vi "basic-speaker.vi"(4 "Cluster":T2, 5 "Period":i64, 6 "Cluster 2":T1, 7 "Lickometer":refnum<vi>, 9 "Speaker in":refnum<vi>, 10 "reference":refnum<vi>, 11 "Cluster in":refnum<vi>) -> (3 "Cluster 3":T1)   [LabVIEW 2015]
uses:
  Device/Methods/Speaker-Play.vi
  <vilib>/Platform/TimedLoop/XDataNode/wakeup.ctl
  <vilib>/Platform/TimedLoop/XDataNode/XDNodeRunTimeDep.lvlib
  <vilib>/Platform/TimedLoop/XDataNode/nitl_modes.ctl
  <vilib>/Platform/TimedLoop/XDataNode/timing_clust.ctl
  <vilib>/platform/TimedLoop/XDataNode/XDataNode.xnode
  Device/Methods/Lickometer-Read.vi
  Rack/Methods/Rack-Refresh.vi
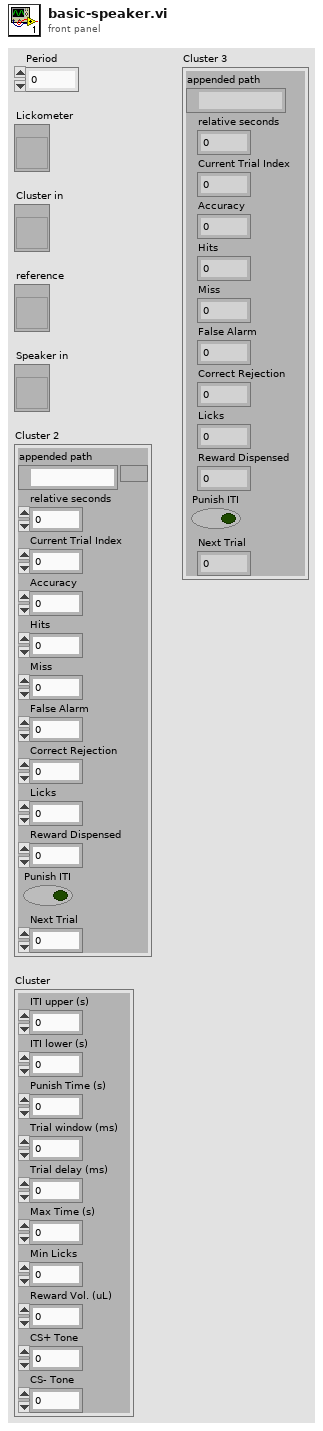
[diagram p1: front panel]
types:
  T1 = cluster{"appended path":path, "relative seconds":dbl, "Current Trial Index":i32, "Accuracy":dbl, "Hits":i32, "Miss":i32, "False Alarm":i32, "Correct Rejection":i32, "Licks":i32, "Reward Dispensed":dbl, "Punish ITI":bool, "Next Trial":i32}
  T2 = cluster{"ITI upper (s)":dbl, "ITI lower (s)":dbl, "Punish Time (s)":dbl, "Trial window (ms)":dbl, "Trial delay (ms)":dbl, "Max Time (s)":dbl, "Min Licks":i32, "Reward Vol. (uL)":dbl, "CS+ Tone":i32, "CS- Tone":i32}
  T3 = typedef "XDNodeRunTimeDep.lvlib/timing_clust.ctl" = cluster{"Expected End [f-1]":u64, "Actual End [f-1]":u64, "Finished Late? [f-1]":bool, "Expected End [i-1]":u64, "Actual End [i-1]":u64, "Finished Late? [i-1]":bool, "Expected Start [i]":u64, "Actual Start [i]":u64, "Expected Start [f]":u64, "Actual Start [f]":u64, "Source Name":string, "Structure Name":string, "Period":i64, "Deadline":i64, "Offset":i64, "Start":i64, "Priority":i32, "Timeout":i32, "Mode":T4, "Wakeup Reason":T5, "Error":errorcluster, "Source Type":string, "Secondary Source Type":string, "Global End Time":u64, "Global Start Time":u64, "Frame Duration":u64, "Iteration Duration":u64, "Assigned CPU":i32, "I/O Scan Engine Mode":u32}
  T4 = typedef "XDNodeRunTimeDep.lvlib/nitl_modes.ctl" = enum32{"No Change", "Process missed periods, maintain original phase", "Discard missed periods, maintain original phase", "Process missed periods, ignore original phase", "Discard missed periods, ignore original phase"}
  T5 = typedef "XDNodeRunTimeDep.lvlib/wakeup.ctl" = enum32{"Normal", "Aborted", "Asynchronous wakeup", "Timing source error", "Timed loop error", "Timeout"}
  T6 = typedef "InputData cluster.ctl" = cluster{"DigitalInput":T7}
  T7 = typedef "DigitalInput-DataCluster.ctl" = cluster{"Falling":bool[], "Rising":bool[], "State":bool[]}
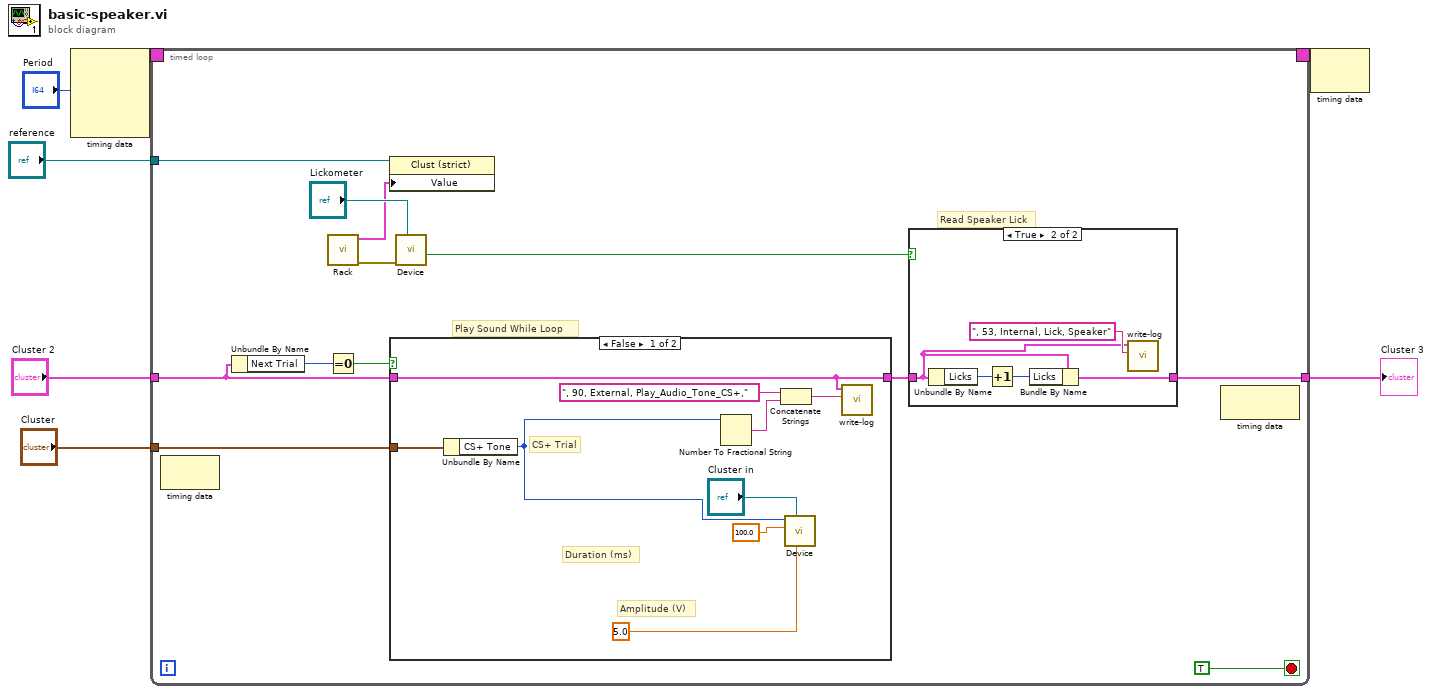
[diagram p0: block diagram]
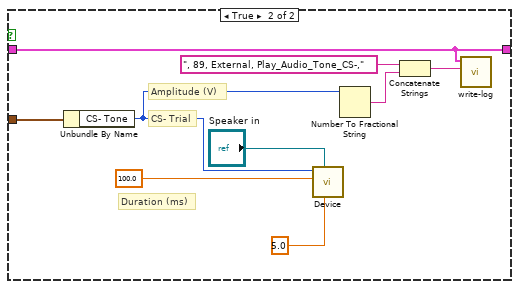
[diagram p3: hidden frame]
diagram:
  n1 = node-c288("Period") -> (w7:T3)  [unwired: 3 in]
  n2 = timed-loop {
    tunnel: "Cluster 2" -> [w17]
    tunnel: [w10] -> w2
    tunnel: "Cluster" -> [w15]
    timing: w7 -> [_]
    timing-out: [_] -> w6
    tunnel: "reference" -> [w8]
    stop <- TRUE stop-if-true
    # "Read Speaker Lick"
    # "Play Sound While Loop"
    n3 = node-c288() -> ()  [unwired: 1 in, 1 out]
    n4 = Unbundle By Name(w17) -> ("Next Trial"=w18:i32)
    n5 = call-poly "Rack.vi"() -> ("error out"=w14:errorcluster, "Data Cluster"=w12:T6)  [unwired: 10 in]
    n6 = Equal To 0?(x=w18) -> (x = 0?=w16:bool)
    n7 = property class="Clust (strict)"(reference=w8, "Value"=w12) -> ()  [unwired: 1 in, 2 out]
    n8 = case shown="False" w16 {
      tunnel: w17 -> [w36 w45]
      tunnel: [w36 w45] -> w11
      tunnel: w15 -> [w35 w41]
      frame False {
        # "Duration (ms)"
        # "Amplitude (V)"
        # "CS+ Trial"
        n9 = Unbundle By Name(w35) -> ("CS+ Tone"=w28:i32)
        n10 = Number To Fractional String(number=w28) -> (F-format string=w34:string)  [unwired: 3 in]
        n11 = Concatenate Strings(", 90, External, Play_Audio_Tone_CS+," ("text"), w34) -> (w32:string)
        n12 = call-poly "Device.vi"("Amplitude (V)"=5.0, "Device reference"="Cluster in", "Duration (ms)"=100.0, "Frequency (Hz)"=w28) -> ()  [unwired: 7 in, 1 out]
        n13 = call "write-log.vi"("Write Text"=w32, "Internal Cluster"=w36) -> ()  [unwired: 10 in]
      }
      frame True {
        # "Duration (ms)"
        # "Amplitude (V)"
        # "CS- Trial"
        n14 = Unbundle By Name(w41) -> ("CS- Tone"=w37:i32)
        n15 = call-poly "Device.vi"("Amplitude (V)"=5.0, "Device reference"="Speaker in", "Duration (ms)"=100.0, "Frequency (Hz)"=w37) -> ()  [unwired: 7 in, 1 out]
        n16 = Number To Fractional String(number=w37) -> (F-format string=w42:string)  [unwired: 3 in]
        n17 = Concatenate Strings(", 89, External, Play_Audio_Tone_CS-," ("text"), w42) -> (w43:string)
        n18 = call "write-log.vi"("Write Text"=w43, "Internal Cluster"=w45) -> ()  [unwired: 10 in]
      }
    }
    n19 = call-poly "Device.vi"("Device reference"="Lickometer", "error in (no error)"=w14) -> ("Lick start?"=w9:bool)  [unwired: 7 in, 2 out]
    n20 = case shown="True" w9 {
      tunnel: w11 -> [w20 w21]
      tunnel: [w20 w25] -> w10
      frame False {
      }
      frame True {
        n21 = Unbundle By Name(w21) -> ("Licks"=w24:i32)
        n22 = Increment(x=w24) -> (x+1=w23:i32)
        n23 = Bundle By Name(cluster=w21, "Licks"=w23) -> (w25:T1)
        n24 = call "write-log.vi"("Write Text"=", 53, Internal, Lick, Speaker" ("text"), "Internal Cluster"=w21) -> ()  [unwired: 10 in]
      }
    }
    n25 = node-c288() -> ()  [unwired: 1 in, 1 out]
  }
  "Cluster 3" <- w2
  n26 = node-c288(w6) -> ()  [unwired: 1 out]
